vi "Get Sensor Serial Number.vi"(8 "Error in (no error)":errorcluster) -> (0 "Error out":errorcluster, 3 "Serial Number":string)   [LabVIEW 2022 SP3]
uses:
  BonTechDetector/BonTechDetector.lvlib
panel:
  out "function return":i32
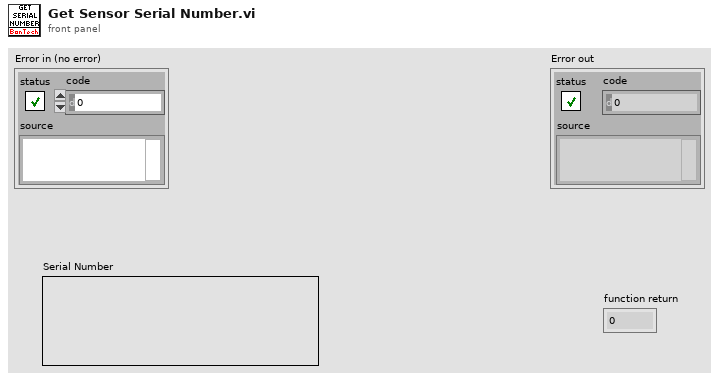
[diagram p1: front panel]
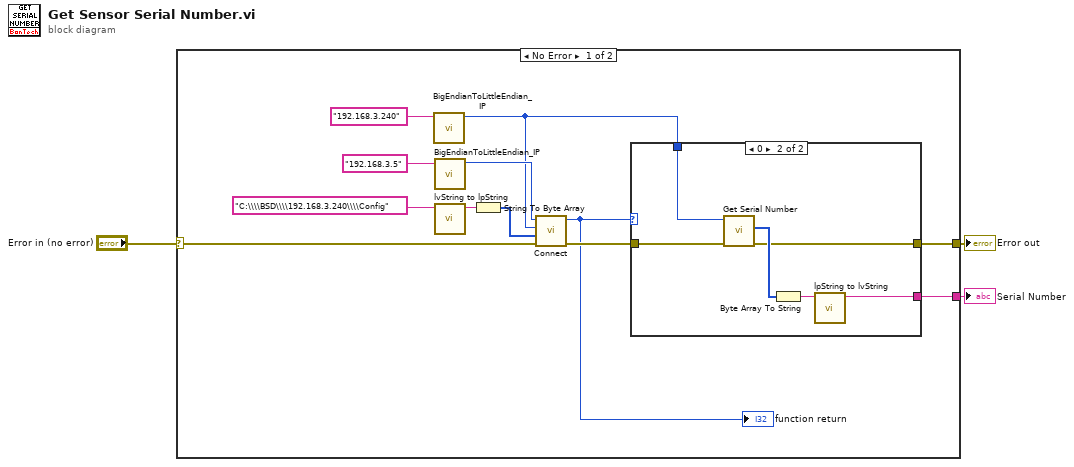
[diagram p0: block diagram]
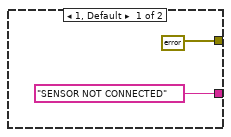
[diagram p2: hidden frame]
diagram:
  n1 = case shown="No Error" "Error in (no error)" {
    selector: "Error in (no error)" -> [w4 w24]
    tunnel: [w14 _] -> w3
    tunnel: [w7 w24] -> w2
    frame No Error {
      n2 = call "BigEndianToLittleEndian_IP.vi"("IP String"="192.168.3.240") -> ("IP Network Order"=w6:u32)  [unwired: 10 in]
      n3 = call "BigEndianToLittleEndian_IP.vi"("IP String"="192.168.3.5") -> ("IP Network Order"=w10:u32)  [unwired: 10 in]
      n4 = call "lvString to lpString.vi"("LVString"="C:\\\\BSD\\\\192.168.3.240\\\\Config" ("IP String")) -> ("LPTSTR String"=w8:string)  [unwired: 10 in]
      n5 = String To Byte Array(string=w8) -> (unsigned byte array=w15:u8[])
      n6 = call "Connect.vi"("error in (no error)"=w4, "ConfigDir"=w15, "nSensorIP"=w6, "nHostIP"=w10) -> ("error out"=w13:errorcluster, "function return"=w5:i32)  [unwired: 6 in]
      "function return" <- w5
      n7 = case shown="0" w5 {
        tunnel: ["SENSOR NOT CONNECTED" ("LVString") w21] -> w14
        tunnel: w13 -> [_ w20]
        tunnel: [errorcluster {"status"=TRUE, "code"=0, "source"=" License Generation Issue! Kindly contact KARMA for support."} ("error out") w18] -> w7
        tunnel: w6 -> [_ w19]
        frame 1, Default {
        }
        frame 0 {
          n8 = call "Get Serial Number.vi"("error in (no error)"=w20, "nSensorIP"=w19) -> ("error out"=w18:errorcluster, "lpszSerialNum out"=w23:u8[])  [unwired: 7 in, 1 out]
          n9 = Byte Array To String(unsigned byte array=w23) -> (string=w22:string)
          n10 = call "lpString to lvString.vi"("LPTSTR String"=w22) -> ("LVString"=w21:string)  [unwired: 10 in]
        }
      }
    }
    frame Error {
    }
  }
  "Serial Number" <- w3
  "Error out" <- w2
